vi "PID.vi"(0 "sp":dbl, 1 "p":dbl, 2 "i":dbl, 3 "d":dbl, 5 "pv":dbl, 7 "maxim":dbl, 9 "minim":dbl) -> (4 "output variable":dbl)   [LabVIEW 2014]
panel:
  out "deriv":dbl
  out "prop":dbl
  out "integ":dbl
  out "err":dbl
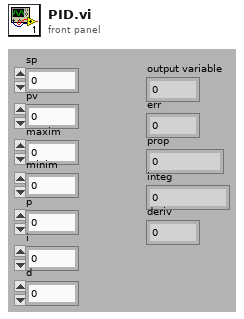
[diagram p1: front panel]
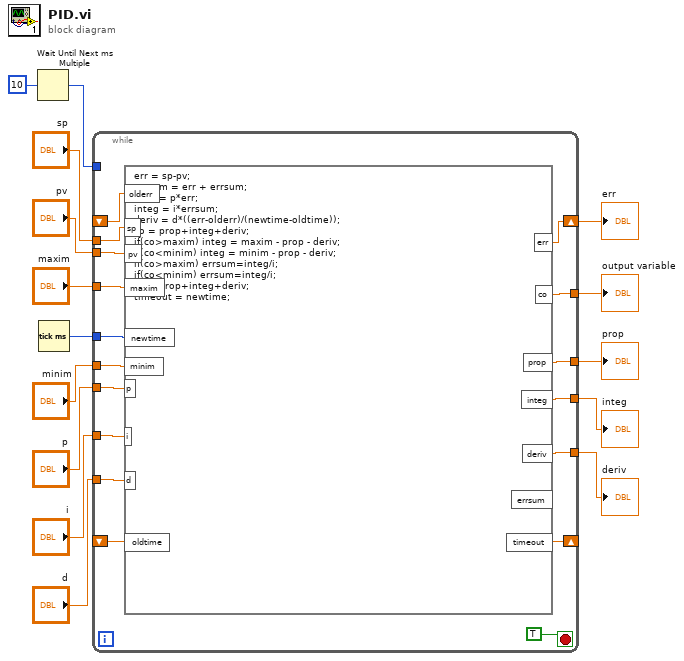
[diagram p0: block diagram]
diagram:
  n1 = Wait Until Next ms Multiple(millisecond multiple=u32 10) -> (millisecond timer value=w2:u32)
  n2 = Tick Count (ms)() -> (millisecond timer value=w8:u32)
  n3 = while {
    tunnel: "sp" -> [w32]
    tunnel: "pv" -> [w31]
    tunnel: "maxim" -> [w30]
    tunnel: "p" -> [w29]
    tunnel: "i" -> [w28]
    tunnel: "d" -> [w27]
    tunnel: "minim" -> [w26]
    tunnel: w8 -> [w25]
    shift-right: [w24] -> w6
    shift-left: _ -> [w23]
    shift-right: [w22] -> _
    shift-left: _ -> [w21]
    tunnel: [w19] -> w7
    tunnel: [w18] -> w5
    tunnel: [w17] -> w4
    tunnel: [w16] -> w3
    tunnel: w2 -> [_]
    stop <- TRUE stop-if-true
    n4 = formula code="err = sp-pv;\nerrsum = err + errsum;\nprop = p*err;\ninteg = i*errsum;\nderiv = d*((err-olderr)/(newtime-oldtime));\nco = prop+integ+deriv;\nif(co>maxim) integ = maxim - prop - deriv;\nif(co<minim) integ = minim - prop - deriv;\nif(co>maxim) errsum=integ/i;\nif(co<minim) errsum=integ/i;\nco = prop+integ+deriv;\ntimeout = newtime;"("sp"=w32, "pv"=w31, "maxim"=w30, "minim"=w26, "p"=w29, "i"=w28, "d"=w27, "olderr"=w23, "newtime"=w25, "oldtime"=w21) -> ("co"=w19:dbl, "err"=w24:dbl, "prop"=w18:dbl, "integ"=w17:dbl, "deriv"=w16:dbl, "timeout"=w22:dbl)  [unwired: 1 out]
  }
  "output variable" <- w7
  "err" <- w6
  "integ" <- w4
  "prop" <- w5
  "deriv" <- w3
